vi "Init Actor.vi"() -> (2 "Actor":refnum<class "Actor.lvclass">)   [LabVIEW 2020, in "jettl.lvlib" / "Base jettl Actor.lvlib" / "Base Actor.lvlib"]
uses:
  Base Actor.lvlib
  Actor/Actor.lvclass
  Base Actor/Base Actor.lvclass
  C:/git/jettl/src/jettl/jettl/Actor/Actor.lvclass
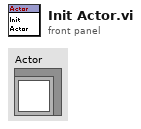
[diagram p1: front panel]
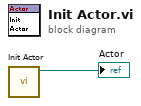
[diagram p0: block diagram]
diagram:
  n1 = call "Init Actor.vi"() -> ("Base Actor out"=→"Actor":refnum<class "Base Actor.lvclass">)  [unwired: 11 in]
